vi "ACal-Draw Multibands.vi"(0 "Fstart":dbl[](array[numeric]), 2 "XYGraph in":refnum<vi>, 7 "Plot":i32) -> ()   [LabVIEW 2020]
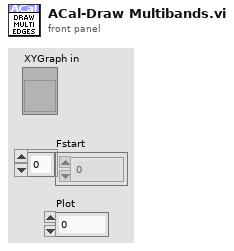
[diagram p1: front panel]
types:
  T1 = typedef "LVRectTypeDef.ctl" = cluster{"Left":i16, "Top":i16, "Right":i16, "Bottom":i16}
  T2 = cluster{"Width":u16, "Style":enum32{"Solid", "Dash", "Dot", "DashDot", "DashDotDot"}}
  T3 = typedef "LVPoint32TypeDef.ctl" = cluster{"Horizontal":i32, "Vertical":i32}
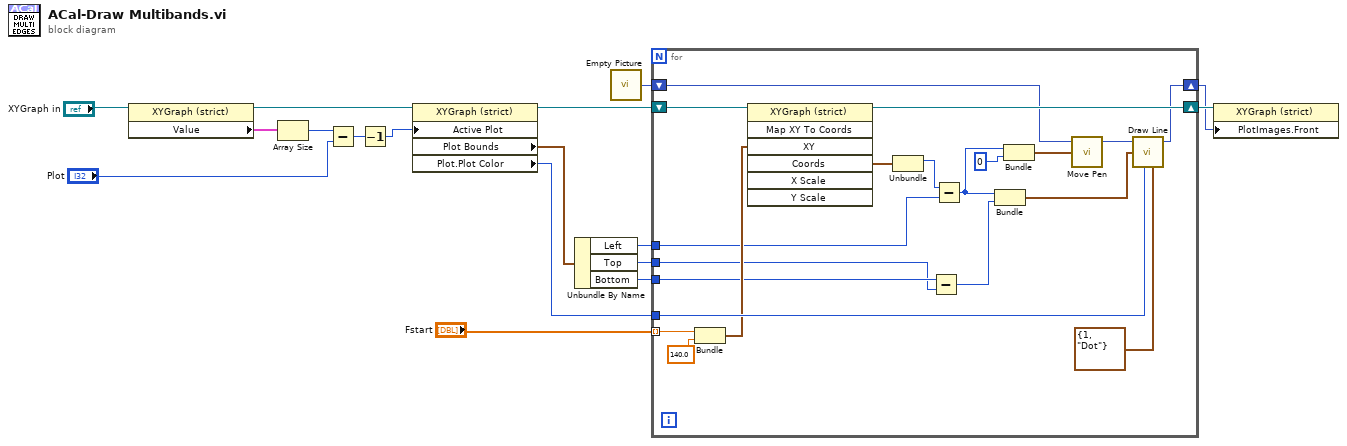
[diagram p0: block diagram]
diagram:
  n1 = property class="XYGraph (strict)"(reference="XYGraph in") -> (reference out=w12:refnum<vi>, "Value"=w16:cluster{"PTC Mag":dbl[], "PTC Phase":dbl[]}[])  [unwired: 1 in, 1 out]
  n2 = Array Size(array=w16) -> (size(s)=w15:i32)
  n3 = Subtract(x=w15, y="Plot") -> (x-y=w13:i32)
  n4 = Decrement(x=w13) -> (x-1=w11:i32)
  n5 = property class="XYGraph (strict)"(reference=w12, "Active Plot"=w11) -> (reference out=w9:refnum<vi>, "Plot Bounds"=w7:T1, "Plot.Plot Color"=w10:u32)  [unwired: 1 in, 1 out]
  n6 = Unbundle By Name(w7) -> ("Left"=w6:i16, "Top"=w4:i16, "Bottom"=w5:i16)
  n7 = call "Empty Picture"() -> ("empty picture"=w3:picture)
  n8 = for {
    tunnel: w10 -> [w36]
    tunnel: w6 -> [w28]
    tunnel: w5 -> [w25]
    tunnel: w4 -> [w21]
    shift-right: [w30] -> w8
    shift-left: w9 -> [w34]
    shift-right: [w19] -> w2
    shift-left: w3 -> [w20]
    tunnel: "Fstart" -> [w18] mode=indexing
    n9 = Bundle("Numeric"=w18, 140.0) -> (w32:cluster{"Numeric":dbl, dbl})  [unwired: 1 in]
    n10 = invoke class="XYGraph (strict)" method="Map XY To Coords"(reference=w34, "XY"=w32) -> (reference out=w30:refnum<vi>, "Coords"=w31:T3)  [unwired: 5 in, 5 out]
    n11 = Unbundle(w31) -> ("Horizontal"=w29:i32)  [unwired: 1 out]
    n12 = Subtract(x=w25, y=w21) -> (x-y=w23:i16)
    n13 = Subtract(x=w29, y=w28) -> (x-y=w26:i32)
    n14 = Bundle(w26, w23) -> (w24:cluster{i32, i16})  [unwired: 1 in]
    n15 = Bundle(w26, 0) -> (w27:cluster{i32, i32})  [unwired: 1 in]
    n16 = call <vilib>:"Move Pen.vi"("new position"=w27, "picture"=w20) -> ("new picture"=w37:picture)  [unwired: 3 in]
    n17 = call <vilib>:"Draw Line.vi"("picture"=w37, "end point"=w24, "color(black)"=w36, "pen"=T2 {"Width"=1, "Style"=enum."Dot"}) -> ("new picture"=w19:picture)  [unwired: 5 in]
  }
  n18 = property class="XYGraph (strict)"(reference=w8, "PlotImages.Front"=w2) -> ()  [unwired: 1 in, 2 out]
